vi "Maximise.vi"(8 "error in (no error)":errorcluster, 9 "Maximised":bool, 11 "module in":refnum<class "TitleBar.lvclass">) -> (0 "error out":errorcluster, 3 "module out":refnum<class "TitleBar.lvclass">)   [LabVIEW 2024, in "TitleBar.lvclass"]
uses:
  TitleBar.lvclass
  TitleBar.lvclass/TitleBar.ctl
  JQMHCore/Module/RQMHModule.lvclass
  Maximise.ctl
  C:/DevOps/CORTEX/JQMH/JQMHCore/Module/RQMHModule.lvclass
  C:/DevOps/CORTEX/JQMH/ModuleTemplates/TitleBar/TitleBar.lvclass
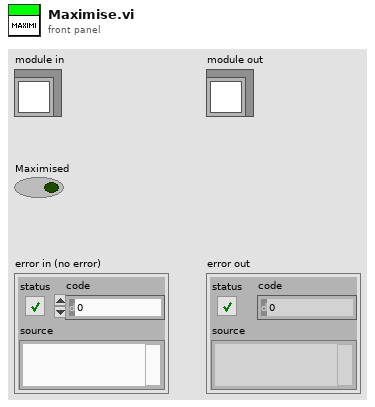
[diagram p1: front panel]
types:
  T1 = typedef "TitleBar.lvclass/Maximise.ctl" = cluster{"Module":refnum<class "RQMHModule.lvclass">, "Maximised":bool}
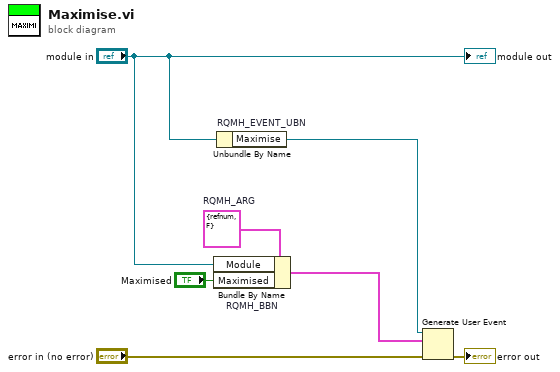
[diagram p0: block diagram]
diagram:
  w4 = T1 {"Module"=refnum, "Maximised"=FALSE}  # RQMH_ARG
  n1 = Bundle By Name "RQMH_BBN"(cluster=w4, "Module"="module in", "Maximised"="Maximised") -> (w3:T1)
  n2 = Unbundle By Name "RQMH_EVENT_UBN"("module in") -> ("Maximise"=w7:refnum<user-event>)
  n3 = Generate User Event(user event=w7, event data cluster=w3, error in="error in (no error)") -> (error out=→"error out":errorcluster)  [unwired: 1 in, 1 out]
  "module out" <- "module in"
